vi "Arttu_v09_99.vi"() -> ()   [LabVIEW 2016]
uses:
  Desktop/Bertta-Bertta_deploy/Bertta-Bertta_deploy/BERTTA/x64/Debug/BERTTA.dll
panel:
  out "element":bool
  out "Started:":string
  in  "SHUTDOWN":bool
  in  "MASTER CONTROL":bool
  in  "Tab Control":T1(tab)
  out "Output File":path caption="selected path"
  in  "Browse folder":path=path "" caption="start path"
  in  "Read Seq":bool
  in  "Save Seq":bool
  in  "Configuration file":path=path "C:/Users/shresplab/Desktop/ArttuConfiguration.lvm" caption="Filename"
  in  "OK Button 2":bool
  out "Boolean":bool
  in  "User (initials)":string
  in  "Project name":string
  in  "Description":string
  out "PUMP1":bool
  out "Target amount":dbl
  out "Scale weight":dbl
  out "Amount now":dbl
  out "Flow rate":dbl
  out "Time to target":dbl format="%<%H:%M:%S>t"
  out "Current step":dbl
  out "Target":dbl
  out "Amount now":dbl
  out "Amount now":dbl
  out "Target":dbl
  out "Current step":dbl
  out "Time to target":dbl format="%<%H:%M:%S>t"
  out "Flow rate":dbl
  out "Amount now":dbl
  out "Scale weight":dbl
  out "Target amount":dbl
  out "PUMP2":bool
  out "Sensor OK 6":bool
  out "Sensor OK 5":bool
  out "Sensor OK 4":bool
  out "Sensor OK 3":bool
  in  "OK Button":bool
  in  "Add comment":string
  out "PUMP3":bool
  out "Target amount":dbl
  out "Scale weight":dbl
  out "Amount now":dbl
  out "Flow rate":dbl
  out "Time to target":dbl format="%<%H:%M:%S>t"
  out "Current step":dbl
  out "Target":dbl
  out "Amount now":dbl
  out "Tr":dbl
  out "Tj in":dbl
  out "Tj out":dbl
  out "T set":dbl
  out "Current step":i32
  out "RPM":dbl
  out "Torque 2":dbl
  out "Waveform Chart 5":dynamicdata(graph)
  out "Waveform Chart 6":dynamicdata(graph)
  out "Waveform Chart 7":dynamicdata(graph)
  in  "Tab Control 2":T2(tab)
  out "Waveform Chart 3":dynamicdata(graph)
  out "Waveform Chart 8":dynamicdata(graph)
  out "Waveform Chart 11":dynamicdata(graph)
  out "Waveform Chart 13":dynamicdata(graph)
  out "Waveform Chart 9":dynamicdata(graph)
  out "Table":string[][](table)=[["14.8.2017 18.06.59", "0,000000", "417,670000", "-0,150000", "1,000000", "22,220000", "23,366837", "23,574959", "23,985852", "23,690000", "240,000000", "4,000000", "0,000000", "397,000000", "-397,000000", "1,000000"], ["14.8.2017 18.07.06", "0,000000", "417,640000", "-0,120000", "1,000000", "22,220000", "23,763115", "23,906257", "23,985694", "23,680000", "240,000000", "4,000000", "0,000000", "397,000000", "-397,000000", "1,000000"], ["14.8.2017 18.07.13", "0,000000", "417,640000", "-0,120000", "1,000000", "22,220000", "23,965922", "24,013440", "23,984906", "23,670000", "240,000000", "4,100000", "3,000000", "397,000000", "-397,000000", "1,000000"], ["14.8.2017 18.07.21", "0,000000", "417,640000", "-0,120000", "1,000000", "22,220000", "23,943860", "23,900110", "23,987113", "23,670000", "240,000000", "4,000000", "0,000000", "397,000000", "-397,000000", "1,000000"], ["14.8.2017 18.07.28", "0,000000", "417,640000", "-0,120000", "1,000000", "22,220000", "23,736328", "23,600018", "23,989004", "23,660000", "240,000000", "4,000000", "0,000000", "397,000000", "-397,000000", "1,000000"], ["14.8.2017 18.07.36", "0,000000", "417,640000", "-0,120000", "1,000000", "22,220000", "23,480910", "23,324538", "23,991053", "23,660000", "240,000000", "4,000000", "0,000000", "397,000000", "-397,000000", "1,000000"], ["14.8.2017 18.07.43", "0,000000", "417,640000", "-0,120000", "2,000000", "22,220000", "23,195579", "23,008270", "23,999093", "23,650000", "240,000000", "4,000000", "0,000000", "397,000000", "-397,000000", "1,000000"], ["14.8.2017 18.07.51", "0,000000", "417,650000", "-417,650000", "1,000000", "22,220000", "22,862541", "22,649021", "24,003979", "23,650000", "240,000000", "4,000000", "0,000000", "397,000000", "-397,000000", "2,000000"], ["14.8.2017 18.07.58", "0,000000", "417,640000", "0,010000", "1,000000", "22,220000", "22,541353", "22,354878", "24,005398", "23,650000", "240,000000", "4,000000", "0,000000", "397,000000", "-397,000000", "1,000000"], ["14.8.2017 18.08.06", "0,000000", "417,640000", "0,010000", "1,000000", "22,220000", "22,347931", "22,253738", "24,007605", "23,640000", "240,000000", "4,100000", "0,000000", "397,000000", "-397,000000", "1,000000"], ["14.8.2017 18.08.13", "0,000000", "417,640000", "0,010000", "1,000000", "22,220000", "22,329030", "22,302102", "24,006028", "23,640000", "240,000000", "4,000000", "0,000000", "395,820000", "-395,820000", "1,000000"], ["14.8.2017 18.08.20", "0,000000", "417,640000", "0,010000", "1,000000", "22,220000", "22,466849", "22,511320", "24,002403", "23,630000", "240,000000", "4,000000", "0,000000", "395,830000", "-0,010000", "1,000000"], ["14.8.2017 18.08.28", "0,000000", "417,640000", "0,010000", "1,000000", "22,220000", "22,707062", "22,835101", "24,000984", "23,620000", "240,000000", "4,000000", "0,000000", "395,830000", "-0,010000", "1,000000"], ["14.8.2017 18.08.35", "0,000000", "417,640000", "0,010000", "1,000000", "22,220000", "23,054104", "23,232979", "24,001299", "23,600000", "240,000000", "4,000000", "0,000000", "395,830000", "-0,010000", "1,000000"], ["14.8.2017 18.08.43", "0,000000", "417,640000", "0,010000", "1,000000", "22,220000", "23,412371", "23,522793", "24,002560", "23,590000", "240,000000", "4,000000", "0,000000", "395,820000", "0,000000", "1,000000"], ["14.8.2017 18.08.51", "0,000000", "417,640000", "0,010000", "1,000000", "22,220000", "23,596247", "23,656125", "24,003821", "23,580000", "240,000000", "4,000000", "0,000000", "395,820000", "0,000000", "1,000000"]]
  in  "Manual/Ramp 3":bool=TRUE
  in  "Manual/Ramp 2":bool=TRUE
  out "Boolean 4":bool
  out "Boolean 3":bool
  out "Boolean 2":bool
  in  "Reset 6":bool
  in  "Manual/Ramp":bool=TRUE
  in  "Array":dbl[][](array[numeric])=[[20.0, 0.0], [20.0, 0.0], [20.0, 0.0]]
  in  "?":bool
  in  "Time":dbl format="Time to target (min):                %#_g"
  out "Current temp":dbl format="Current temperature (S1):   %#_6g"
  in  "OK Button 3":bool
  out "Sensor OK":bool
  in  "T fail":dbl=20.0 format="Failsafe temperature:              %#_g"
  in  "Setpoint":dbl=20.0 format="Temperature target:                %#_6g"
  out "Waveform Chart":dynamicdata(graph)
  out "T external 2":dbl format="Current temp (S2):    %#_g"
  in  "UPDATE TEMP":bool
  out "Led11 5":bool
  out "RPM":dbl format="%_4f"
  out "Led10 3":bool
  out "Led9 3":bool
  out "Led8 3":bool
  out "Led7 3":bool
  out "Led6 3":bool
  out "Led5 3":bool
  out "Led4 3":bool
  out "Led3 3":bool
  out "Led2 3":bool
  out "Led1 3":bool
  in  "PumpSeq 4":dbl[][](array[numeric])=[[0.0, 0.0, 0.0, 0.0, 0.0, 0.0, 0.0, 0.0, 0.0, 0.0], [0.0, 0.0, 0.0, 0.0, 0.0, 0.0, 0.0, 0.0, 0.0, 0.0], [0.0, 0.0, 0.0, 0.0, 0.0, 0.0, 0.0, 0.0, 0.0, 0.0], [0.0, 0.0, 0.0, 0.0, 0.0, 0.0, 0.0, 0.0, 0.0, 0.0], [0.0, 0.0, 0.0, 0.0, 0.0, 0.0, 0.0, 0.0, 0.0, 0.0], [0.0, 0.0, 0.0, 0.0, 0.0, 0.0, 0.0, 0.0, 0.0, 0.0], [0.0, 0.0, 0.0, 0.0, 0.0, 0.0, 0.0, 0.0, 0.0, 0.0], [0.0, 0.0, 0.0, 0.0, 0.0, 0.0, 0.0, 0.0, 0.0, 0.0], [0.0, 0.0, 0.0, 0.0, 0.0, 0.0, 0.0, 0.0, 0.0, 0.0], [0.0, 0.0, 0.0, 0.0, 0.0, 0.0, 0.0, 0.0, 0.0, 0.0]]
  in  "?":bool
  out "Flow rate (g/min)":dbl
  out "Scale reading":dbl
  out "Step amount now":dbl
  in  "Grams / min":dbl
  out "Waveform Chart 14":dynamicdata(graph)
  in  "?":bool
  out "Total amount now":dbl
  out "Led11 4":bool
  in  "Reset 5":bool
  out "Elapsed / step":i32
  out "Time to target":dbl format="%<%H:%M:%S>t"
  in  "OK Button 4":bool
  out "Led11":bool
  out "RPM":dbl format="%_4f"
  out "Led10":bool
  out "Led9":bool
  out "Led8":bool
  out "Led7":bool
  out "Led6":bool
  out "Led5":bool
  out "Led4":bool
  out "Led3":bool
  out "Led2":bool
  out "Led1":bool
  in  "PumpSeq 2":dbl[][](array[numeric])=[[0.0, 0.0, 0.0, 0.0, 0.0, 0.0, 0.0, 0.0, 0.0, 0.0], [0.0, 0.0, 0.0, 0.0, 0.0, 0.0, 0.0, 0.0, 0.0, 0.0], [0.0, 0.0, 0.0, 0.0, 0.0, 0.0, 0.0, 0.0, 0.0, 0.0], [0.0, 0.0, 0.0, 0.0, 0.0, 0.0, 0.0, 0.0, 0.0, 0.0], [0.0, 0.0, 0.0, 0.0, 0.0, 0.0, 0.0, 0.0, 0.0, 0.0], [0.0, 0.0, 0.0, 0.0, 0.0, 0.0, 0.0, 0.0, 0.0, 0.0], [0.0, 0.0, 0.0, 0.0, 0.0, 0.0, 0.0, 0.0, 0.0, 0.0], [0.0, 0.0, 0.0, 0.0, 0.0, 0.0, 0.0, 0.0, 0.0, 0.0], [0.0, 0.0, 0.0, 0.0, 0.0, 0.0, 0.0, 0.0, 0.0, 0.0], [0.0, 0.0, 0.0, 0.0, 0.0, 0.0, 0.0, 0.0, 0.0, 0.0]]
  in  "?":bool
  out "Flow rate (g/min)":dbl
  out "Scale reading":dbl
  out "Step amount now":dbl
  in  "Grams / min":dbl
  out "Waveform Chart 10":dynamicdata(graph)
  in  "?":bool
  out "Total amount now":dbl
  out "Led11":bool
  in  "Reset 3":bool
  out "Elapsed / step":i32
  out "Time to target":dbl format="%<%H:%M:%S>t"
  in  "OK Button 5":bool
  out "Led11 3":bool
  out "RPM":dbl format="%_4f"
  out "Led10 2":bool
  out "Led9 2":bool
  out "Led8 2":bool
  out "Led7 2":bool
  out "Led6 2":bool
  out "Led5 2":bool
  out "Led4 2":bool
  out "Led3 2":bool
  out "Led2 2":bool
  out "Led1 2":bool
  in  "PumpSeq 3":dbl[][](array[numeric])=[[0.0, 0.0, 0.0, 0.0, 0.0, 0.0, 0.0, 0.0, 0.0, 0.0], [0.0, 0.0, 0.0, 0.0, 0.0, 0.0, 0.0, 0.0, 0.0, 0.0], [0.0, 0.0, 0.0, 0.0, 0.0, 0.0, 0.0, 0.0, 0.0, 0.0], [0.0, 0.0, 0.0, 0.0, 0.0, 0.0, 0.0, 0.0, 0.0, 0.0], [0.0, 0.0, 0.0, 0.0, 0.0, 0.0, 0.0, 0.0, 0.0, 0.0], [0.0, 0.0, 0.0, 0.0, 0.0, 0.0, 0.0, 0.0, 0.0, 0.0], [0.0, 0.0, 0.0, 0.0, 0.0, 0.0, 0.0, 0.0, 0.0, 0.0], [0.0, 0.0, 0.0, 0.0, 0.0, 0.0, 0.0, 0.0, 0.0, 0.0], [0.0, 0.0, 0.0, 0.0, 0.0, 0.0, 0.0, 0.0, 0.0, 0.0], [0.0, 0.0, 0.0, 0.0, 0.0, 0.0, 0.0, 0.0, 0.0, 0.0]]
  in  "?":bool
  out "Flow rate (g/min)":dbl
  out "Scale reading":dbl
  out "Step amount now":dbl
  in  "Grams / min":dbl
  out "Waveform Chart 12":dynamicdata(graph)
  in  "?":bool
  out "Total amount now":dbl
  out "Led11 2":bool
  in  "Reset 4":bool
  out "Elapsed / step":i32
  out "Time to target":dbl format="%<%H:%M:%S>t"
  in  "OK Button 6":bool
  in  "?":bool
  in  "Scale port":dbl=3.0
  out "Waveform Chart 15":dynamicdata(graph)
  in  "?":bool
  in  "OK Button 8":bool
  in  "Remote / Manual":bool
  in  "Set RPM":i32
  out "RPM":dbl
  out "Torque":dbl
  out "Waveform Chart 4":dynamicdata(graph)
  in  "OK Button 7":bool
  out "PortDev out":dbl[](array[numeric])
  in  "Save PortDev":bool
  out "PortDev in":dbl[](array[numeric])
  in  "dev1":i32=1
  in  "dev2":i32=2
  in  "dev3":i32=3
  in  "dev4":i32=4
  in  "dev5":i32=5
  in  "dev6":i32=5
  in  "dev8":i32
  in  "port1":i32=7
  in  "port2":i32=7
  in  "port3":i32=2
  in  "port4":i32=2
  in  "port5":i32=5
  in  "port6":i32=4
  in  "port7":i32=3
  in  "port8":i32
  in  "dev7":i32=5
  in  "Treshold (T/C)":dbl=0.5
  out "DAQ 9217 (PT100)":errorcluster
  out "Config File":dbl[][](array[numeric])
  in  "Temp Control":tag="cDAQ9188XT-1C3BEFEMod1"
  in  "PAM Control":tag="cDAQ9188XT-1C3BEFEMod7"
  # "Temperature sensor:"
  # "Manual control:"
  # "PUMP & SCALE 1"
  # "STEP"
  # "TOTAL"
  # "PUMP & SCALE 2"
  # "STEP"
  # "TOTAL"
  # "PUMP & SCALE 3"
  # "STEP"
  # "TOTAL"
  # "Temperature control parameter"
  # "Secondary temperature sensor"
  # "Temp target"
  # "Time target"
  # "Grams    /   min"
  # "End of sequence"
  # "Manual control"
  # "Grams    /   min"
  # "End of sequence"
  # "Manual control"
  # "Grams    /   min"
  # "End of sequence"
  # "Manual control"
  # "PAM control"
  # "dev1 and dev2 always to port1 and 2\nport1 = port2 = Lauda\n\ndev3 and dev4 always to port3 and port4\nport3 = port4 = Heidolph"
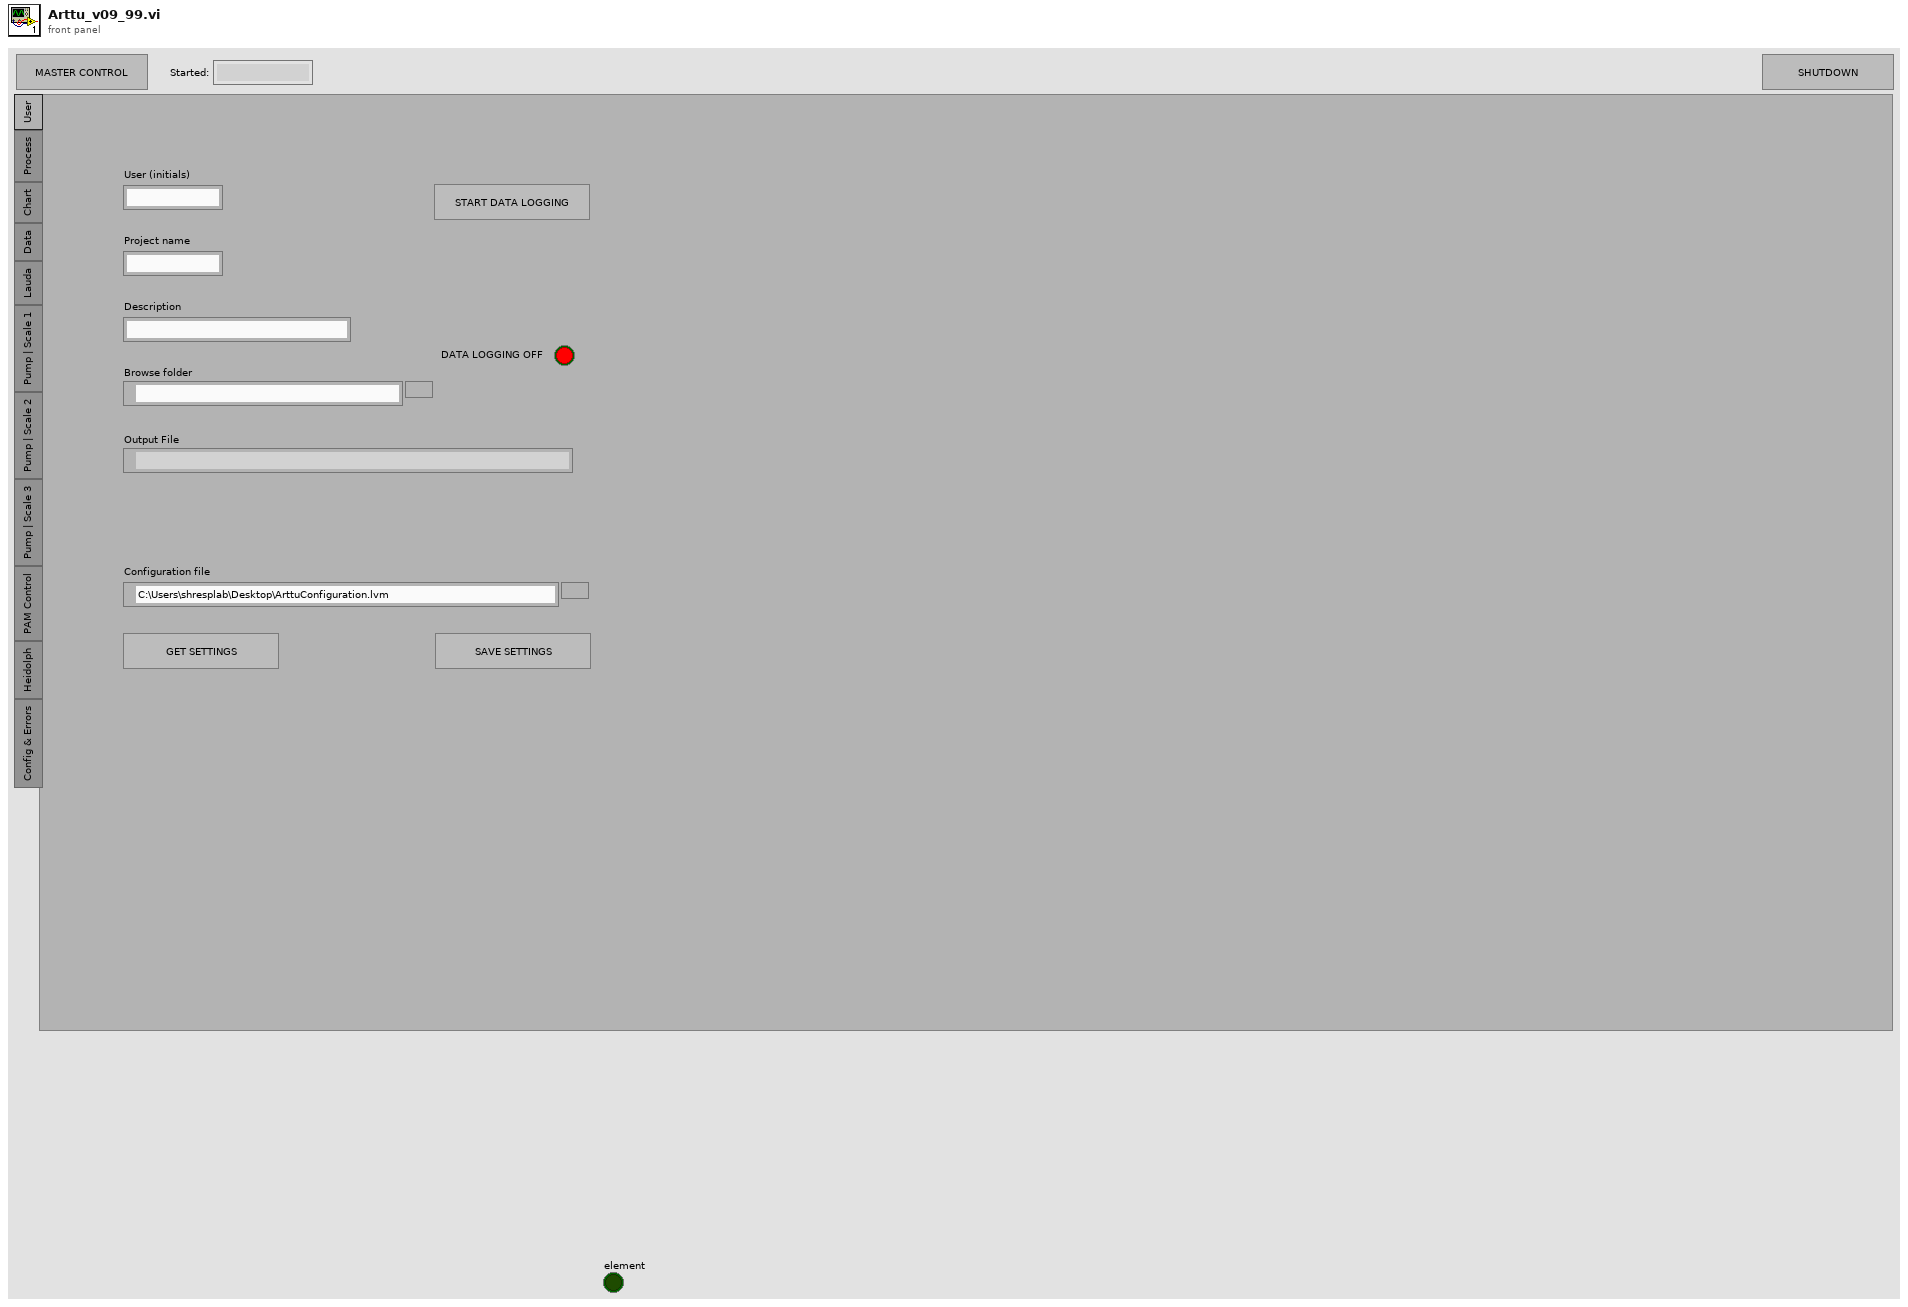
[diagram p1: front panel]
types:
  T1 = enum32{"User", "Process", "Chart", "Data", "Lauda", "Pump | Scale 1", "Pump | Scale 2", "Pump | Scale 3", "PAM Control", "Heidolph", "Config & Errors"}
  T2 = enum32{"Temperatures", "Scale / Pump 1", "Scale / Pump 2", "Scale / Pump 3", "RPM / torque"}
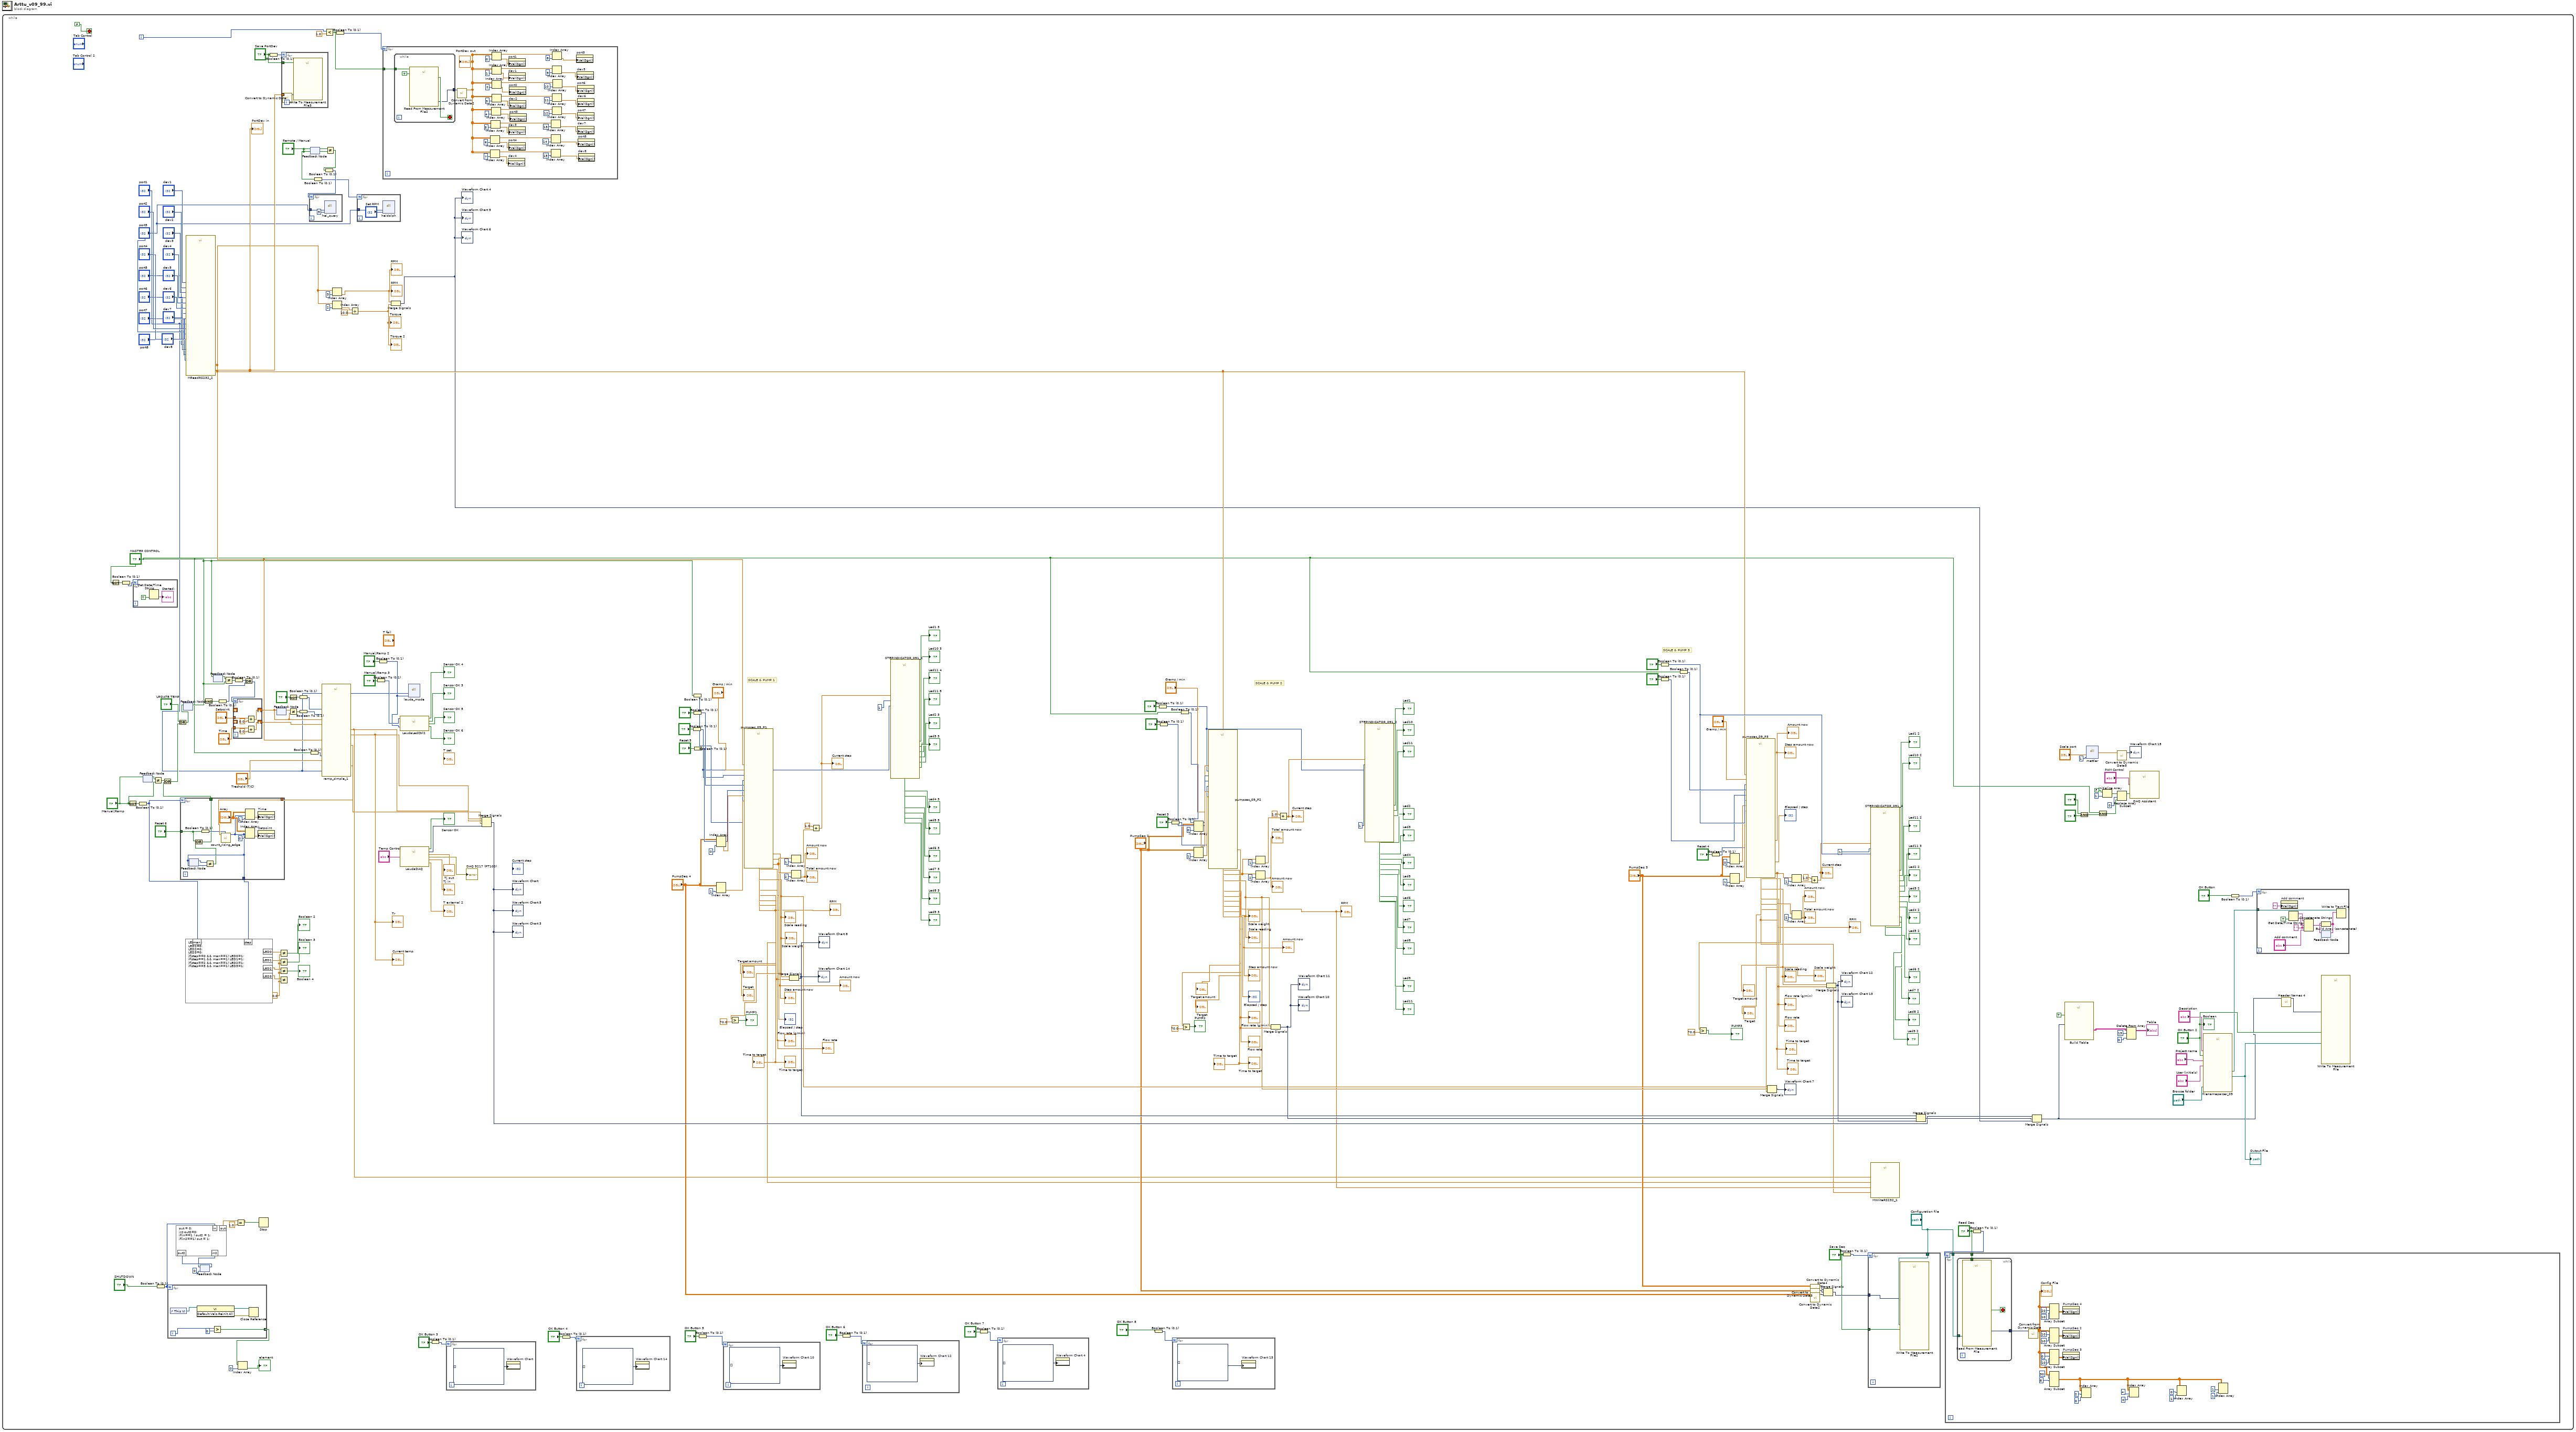
[diagram p0: block diagram]
diagram:
  n1 = while {
    i -> [w65]
    stop <- FALSE stop-if-true
    w51 = 0.0 ("y")
    # "SCALE & PUMP 1"
    # "SCALE & PUMP 3"
    # "SCALE & PUMP 2"
    n2 = Not(x="MASTER CONTROL") -> (.not. x?=w292:bool)
    n3 = Boolean To (0,1)(Boolean=w292) -> (0, 1=w293:i16)
    n4 = Not(x="Manual/Ramp") -> (.not. x?=w58:bool)
    n5 = for {
      N: w293 -> [_]
      n6 = Get Date/Time String(want seconds? (F)=TRUE) -> (time string=→"Started:":string)  [unwired: 2 in, 1 out]
    }
    n7 = Boolean To (0,1)(Boolean=w58) -> (0, 1=w40:i16)
    n8 = feedback #1() -> (w46:bool)  [unwired: 1 in]
    n9 = feedback-in #1("Manual/Ramp") -> ()
    n10 = Not Equal?(x=w46, y="Manual/Ramp") -> (x != y?=w43:bool)
    n11 = Boolean To (0,1)(Boolean="SHUTDOWN") -> (0, 1=w277:i16)
    n12 = for {
      N: w277 -> [_]
      tunnel: [w409] -> w291 mode=indexing
      i -> [w411]
      n13 = control-ref of="This VI"() -> (w414:refnum<vi>)
      n14 = invoke class="VI" method="Default Vals.Reinit All"(reference=w414) -> (reference out=w412:refnum<vi>, error out=w413:errorcluster)  [unwired: 2 in, 1 out]
      n15 = Greater?(x=w411, y=0) -> (0:w409:bool)
      n16 = Close Reference(reference=w412, error in (no error)=w413) -> ()  [unwired: 1 out]
    }
    n17 = feedback #2() -> (w38:bool)  [unwired: 1 in]
    n18 = call "MReadRS232_2.vi"("port1"="port1", "dev1"="dev1", "port2"="port2", "dev2"="dev2", "port3"="port3", "dev7"="dev7", "dev8"="dev8", "port7"="port7", "port8"="port8", "dev5"="dev5", "port5"="port5", "dev4"="dev4", "dev6"="dev6", "port6"="port6", "port4"="port4", "dev3"="dev3") -> ("output array"=w69:dbl[], "params"=w30:dbl[])  [unwired: 2 in]
    "PortDev in" <- w69
    n19 = feedback #3(0) -> (w275:i32)
    n20 = formula code="out = 0;\nint out2=0;\nif(in==1 ) out2 = 1;\nif(in2==1) out = 1;"("in"=w277, "in2"=w275) -> ("out"=w279:dbl, "out2"=w276:i32)
    n21 = feedback-in #3(w276) -> ()
    n22 = And(x="MASTER CONTROL", y=w38) -> (x .and. y?=w96:bool)
    n23 = feedback #4() -> (w87:bool)  [unwired: 1 in]
    n24 = feedback-in #4("MASTER CONTROL") -> ()
    n25 = Boolean To (0,1)(Boolean=w96) -> (0, 1=w85:i16)
    n26 = Not Equal?(x=w87, y="MASTER CONTROL") -> (x != y?=w86:bool)
    n27 = Boolean To (0,1)(Boolean=w86) -> (0, 1=w84:i16)
    n28 = Equal?(x=w279, y=1.0) -> (x = y?=w278:bool)
    n29 = Index Array(array=w291, index=0) -> (element=→"element":bool)
    n30 = Or(x=w84, y=w85) -> (x .or. y?=w83:i16)
    n31 = for {
      N: w83 -> [_]
      tunnel: "Time" -> [w361]
      shift-right: [w360] -> w97
      shift-left: _ -> [_]
      tunnel: "Setpoint" -> [w358]
      shift-right: [w357] -> w94
      shift-left: _ -> [_]
      n32 = Add(x=w358, y=0.0) -> (x+y=w357:dbl)
      n33 = Add(x=w361, y=0.0) -> (x+y=w360:dbl)
    }
    n34 = Stop(stop? (T)=w278) -> ()
    n35 = Boolean To (0,1)(Boolean="Save PortDev") -> (0, 1=w68:i16)
    n36 = feedback-in #5(w94) -> ()
    n37 = feedback #5() -> (w95:dbl)  [unwired: 1 in]
    n38 = for {
      N: w68 -> [_]
      tunnel: w69 -> [w356]
      tunnel: "Save PortDev" -> [w354]
      n39 = call "Convert to Dynamic Data"("Array"=w356) -> ("Dynamic Data Type"=w355:dynamicdata)  [unwired: 3 in]
      n40 = call "Write To Measurement File3"("Signals"=w355, "Reset"=w354) -> ()  [unwired: 15 in, 3 out]
    }
    n41 = Not(x="?") -> (.not. x?=w90:bool)
    n42 = Not Equal?(x=w95, y=w94) -> (x != y?=w93:bool)
    n43 = Boolean To (0,1)(Boolean=w90) -> (0, 1=w92:i16)
    n44 = Boolean To (0,1)(Boolean=w93) -> (0, 1=w88:i16)
    n45 = Boolean To (0,1)(Boolean="MASTER CONTROL") -> (0, 1=w89:i16)
    n46 = feedback-in #6("Remote / Manual") -> ()
    n47 = feedback #6() -> (w35:bool)  [unwired: 1 in]
    n48 = Boolean To (0,1)(Boolean="Remote / Manual") -> (0, 1=w33:i16)
    n49 = call "ramp_simple_1.vi"("pause"=w92, "time_set"=w97, "array"=w30, "reset"=w88, "master"=w89, "T_sp"=w94, "treshold"="Treshold (T/C)", "port"="port1") -> ("Tin"=w100:dbl, "Tr"=w101:dbl, "target_reached"=w56:dbl, "T control"=w102:dbl)  [unwired: 3 in, 1 out]
    "Tr" <- w101
    "Current temp" <- w101
    n50 = for {
      N: w40 -> [_]
      tunnel: w56 -> [w313]
      tunnel: [w303] -> w44
      tunnel: "Reset 6" -> [w305]
      tunnel: [w306] -> w47
      n51 = feedback #7() -> (w307:i32)  [unwired: 1 in]
      n52 = Boolean To (0,1)(Boolean=w305) -> (0, 1=w308:i16)
      n53 = call "count_rising_edge.vi"("reset"=w308, "target_reached"=w313) -> ("element 2"=w306:i32)  [unwired: 9 in]
      n54 = feedback-in #7(w306) -> ()
      n55 = Not Equal?(x=w307, y=w306) -> (x != y?=w304:bool)
      n56 = Or(x=w305, y=w304) -> (x .or. y?=w303:bool)
      n57 = Index Array(array="Array", index (row)=w306, index (col)=1 ("disabled index (col)")) -> (element=w309:dbl)
      n58 = Index Array(array="Array", index (row)=w306, index (col)=0 ("disabled index (col)")) -> (element=w310:dbl)
      n59 = property on="Time" class="DigNum (strict)"("Val(Sgnl)"=w309) -> ()  [unwired: 2 in, 2 out]
      n60 = property on="Setpoint" class="DigNum (strict)"("Val(Sgnl)"=w310) -> ()  [unwired: 2 in, 2 out]
    }
    n61 = Or(x=w43, y=w44) -> (x .or. y?=w42:bool)
    n62 = Or(x="UPDATE TEMP", y=w42) -> (x .or. y?=w39:bool)
    n63 = feedback-in #2(w39) -> ()
    n64 = formula code="LED0=0;\nLED1=0;\nLED2=0;\nLED3=0;\nif(step==0 && man==1) LED0=1;\nif(step==1 && man==1) LED1=1;\nif(step==2 && man==1) LED2=1;\nif(step==3 && man==1) LED3=1;"("step"=w47, "man"=w40) -> ("LED0"=w55:dbl, "LED1"=w54:dbl, "LED2"=w53:dbl, "LED3"=w52:dbl)
    n65 = Not Equal?(x=w55, y=w51) -> (x != y?=→"Boolean 2":bool)
    n66 = Not Equal?(x=w54, y=w51) -> (x != y?=→"Boolean 3":bool)
    n67 = Not Equal?(x=w53, y=w51) -> (x != y?=→"Boolean 4":bool)
    n68 = Not Equal?(x=w52, y=w51) -> ()  [unwired: 1 out]
    n69 = Less?(x=w65, y=1.0) -> (x < y?=w63:bool)
    n70 = Not Equal?(x=w35, y="Remote / Manual") -> (x != y?=w34:bool)
    n71 = Boolean To (0,1)(Boolean=w34) -> (0, 1=w36:i16)
    n72 = for {
      N: w36 -> [_]
      tunnel: "port3" -> [w301]
      n73 = dll-call lib="C:/Users/shresplab/Desktop/Bertta-Bertta_deploy/Bertta-Bertta_deploy/BERTTA/x64/Debug/BERTTA.dll" fn="hei_query"("port"=w301, "q"=5) -> ()  [unwired: 6 in, 2 out]
    }
    n74 = Index Array(array=w30, index=3) -> (element=w27:dbl)
    "RPM" <- w27
    "RPM" <- w27
    n75 = Index Array(array=w30, index=2) -> (element=w29:dbl)
    n76 = Boolean To (0,1)(Boolean=w63) -> (0, 1=w64:i16)
    n77 = Divide(x=w29, y=10.0) -> (x/y=w26:dbl)
    "Torque" <- w26
    "Torque 2" <- w26
    n78 = for {
      N: w33 -> [_]
      tunnel: "port3" -> [w299]
      n79 = dll-call lib="C:/Users/shresplab/Desktop/Bertta-Bertta_deploy/Bertta-Bertta_deploy/BERTTA/x64/Debug/BERTTA.dll" fn="heidolph"("port"=w299, "speed"="Set RPM") -> ()  [unwired: 6 in, 2 out]
    }
    n80 = Boolean To (0,1)(Boolean="Manual/Ramp 3") -> (0, 1=w3:i16)
    n81 = Boolean To (0,1)(Boolean="Manual/Ramp 2") -> (0, 1=w1:i16)
    n82 = for {
      N: w64 -> [_]
      tunnel: w63 -> [w349]
      n83 = while {
        tunnel: [w352] -> w348
        tunnel: w349 -> [w350]
        stop <- w353 stop-if-true
        n84 = call "Read From Measurement File2"("Enable"=TRUE, "Reset"=w350) -> ("Signals"=w352:dynamicdata, "EOF?"=w353:bool)  [unwired: 4 in, 4 out]
      }
      n85 = call "Convert from Dynamic Data2"("Dynamic Data Type"=w348) -> ("Array"=w331:dbl[])  [unwired: 3 in]
      "PortDev out" <- w331
      n86 = Index Array(array=w331, index=6) -> (element=w324:dbl)
      n87 = Index Array(array=w331, index=7) -> (element=w323:dbl)
      n88 = Index Array(array=w331, index=5) -> (element=w325:dbl)
      n89 = Index Array(array=w331, index=4) -> (element=w326:dbl)
      n90 = Index Array(array=w331, index=0) -> (element=w330:dbl)
      n91 = Index Array(array=w331, index=1) -> (element=w329:dbl)
      n92 = Index Array(array=w331, index=3) -> (element=w327:dbl)
      n93 = Index Array(array=w331, index=2) -> (element=w328:dbl)
      n94 = property on="dev4" class="DigNum (strict)"("Val(Sgnl)"=w323) -> ()  [unwired: 2 in, 2 out]
      n95 = property on="dev3" class="DigNum (strict)"("Val(Sgnl)"=w325) -> ()  [unwired: 2 in, 2 out]
      n96 = property on="port4" class="DigNum (strict)"("Val(Sgnl)"=w324) -> ()  [unwired: 2 in, 2 out]
      n97 = property on="port1" class="DigNum (strict)"("Val(Sgnl)"=w330) -> ()  [unwired: 2 in, 2 out]
      n98 = property on="dev1" class="DigNum (strict)"("Val(Sgnl)"=w329) -> ()  [unwired: 2 in, 2 out]
      n99 = property on="port2" class="DigNum (strict)"("Val(Sgnl)"=w328) -> ()  [unwired: 2 in, 2 out]
      n100 = property on="dev2" class="DigNum (strict)"("Val(Sgnl)"=w327) -> ()  [unwired: 2 in, 2 out]
      n101 = property on="port3" class="DigNum (strict)"("Val(Sgnl)"=w326) -> ()  [unwired: 2 in, 2 out]
      n102 = Index Array(array=w331, index=14) -> (element=w316:dbl)
      n103 = Index Array(array=w331, index=15) -> (element=w315:dbl)
      n104 = Index Array(array=w331, index=13) -> (element=w317:dbl)
      n105 = Index Array(array=w331, index=12) -> (element=w318:dbl)
      n106 = Index Array(array=w331, index=8) -> (element=w322:dbl)
      n107 = Index Array(array=w331, index=9) -> (element=w321:dbl)
      n108 = Index Array(array=w331, index=11) -> (element=w319:dbl)
      n109 = Index Array(array=w331, index=10) -> (element=w320:dbl)
      n110 = property on="port5" class="DigNum (strict)"("Val(Sgnl)"=w322) -> ()  [unwired: 2 in, 2 out]
      n111 = property on="dev5" class="DigNum (strict)"("Val(Sgnl)"=w321) -> ()  [unwired: 2 in, 2 out]
      n112 = property on="port6" class="DigNum (strict)"("Val(Sgnl)"=w320) -> ()  [unwired: 2 in, 2 out]
      n113 = property on="dev6" class="DigNum (strict)"("Val(Sgnl)"=w319) -> ()  [unwired: 2 in, 2 out]
      n114 = property on="port7" class="DigNum (strict)"("Val(Sgnl)"=w318) -> ()  [unwired: 2 in, 2 out]
      n115 = property on="dev7" class="DigNum (strict)"("Val(Sgnl)"=w317) -> ()  [unwired: 2 in, 2 out]
      n116 = property on="port8" class="DigNum (strict)"("Val(Sgnl)"=w316) -> ()  [unwired: 2 in, 2 out]
      n117 = property on="dev8" class="DigNum (strict)"("Val(Sgnl)"=w315) -> ()  [unwired: 2 in, 2 out]
    }
    n118 = Merge Signals(w27, w26) -> (w25:dynamicdata)
    "Waveform Chart 4" <- w25
    "Waveform Chart 6" <- w25
    "Waveform Chart 9" <- w25
    n119 = call "LaudaLedCtrl2.vi"("ctrl_mode"=w1, "T ext / T ext in"=w3) -> ("Sensor OK 5"=→"Sensor OK 5":bool, "Sensor OK 3"=→"Sensor OK 3":bool, "Sensor OK 4"=→"Sensor OK 4":bool, "Sensor OK 6"=→"Sensor OK 6":bool)  [unwired: 6 in]
    n120 = call "LaudaDAQ.vi"("device name"="Temp Control") -> ("error out"=→"DAQ 9217 (PT100)":errorcluster, 1:"Tj out"=→"Tj out":dbl, "data"=w169:dynamicdata, "Sensor OK"=→"Sensor OK":bool, 4:"Tj out"=→"Tj in":dbl, "T external 2"=→"T external 2":dbl)  [unwired: 5 in]
    n121 = dll-call lib="C:/Users/shresplab/Desktop/Bertta-Bertta_deploy/Bertta-Bertta_deploy/BERTTA/x64/Debug/BERTTA.dll" fn="lauda_mode"("port"="port1", "mode"=w1) -> ()  [unwired: 6 in, 2 out]
    n122 = Boolean To (0,1)(Boolean="OK Button 3") -> (0, 1=w113:i16)
    n123 = for {
      N: w113 -> [_]
      n124 = property on="Waveform Chart" class="WFChart (strict)"("History Data"=dynamicdata[] []) -> ()  [unwired: 2 in, 2 out]
    }
    n125 = Merge Signals(w102, w101, w100, w169) -> (w170:dynamicdata)
    "Waveform Chart 3" <- w170
    "Waveform Chart" <- w170
    "Waveform Chart 5" <- w170
    n126 = Boolean To (0,1)(Boolean="OK Button 4") -> (0, 1=w111:i16)
    n127 = for {
      N: w111 -> [_]
      n128 = property on="Waveform Chart 14" class="WFChart (strict)"("History Data"=dynamicdata[] []) -> ()  [unwired: 2 in, 2 out]
    }
    n129 = Boolean To (0,1)(Boolean="?") -> (0, 1=w178:i16)
    n130 = Boolean To (0,1)(Boolean="?") -> (0, 1=w182:i16)
    n131 = Boolean To (0,1)(Boolean="MASTER CONTROL") -> (0, 1=w174:i16)
    n132 = Boolean To (0,1)(Boolean="Reset 5") -> (0, 1=w181:i16)
    n133 = Boolean To (0,1)(Boolean="OK Button 5") -> (0, 1=w109:i16)
    n134 = Index Array(array="PumpSeq 4", index (col)=0) -> (element=w186:dbl[])  [unwired: 1 in]
    n135 = Index Array(array="PumpSeq 4", index (col)=1) -> (element=w207:dbl[])  [unwired: 1 in]
    n136 = for {
      N: w109 -> [_]
      n137 = property on="Waveform Chart 10" class="WFChart (strict)"("History Data"=dynamicdata[] []) -> ()  [unwired: 2 in, 2 out]
    }
    n138 = call "pumpsec_09_P1.vi"("reset"=w181, "master"=w174, "manual"=w178, "pause"=w182, "Array"=w30, "Target"=w186, "fr_manual"="Grams / min", "Time"=w207) -> ("pumpCtrl"=w153:dbl, "totaltarget"=→"Target":dbl, "target_step"=→"Target amount":dbl, "REGLO D"=w119:dbl, "time_to_target"=→"Time to target" →"Time to target":dbl, "step_fr"=w130:dbl, "amount_step"=→"Amount now" →"Step amount now":dbl, "Scale"=w165:dbl, "elapsed_step"=→"Elapsed / step":dbl, "params"=w204:dbl[])  [unwired: 8 in, 2 out]
    "Flow rate" <- w130
    "Scale weight" <- w165
    "Scale reading" <- w165
    "Flow rate (g/min)" <- w130
    "RPM" <- w119
    n139 = Greater?(x=w153, y=70.0) -> (0:→"PUMP1":bool)
    n140 = Merge Signals(w165, w130) -> (w173:dynamicdata)
    "Waveform Chart 8" <- w173
    "Waveform Chart 14" <- w173
    n141 = Index Array(array=w204, index=1) -> (element=w201:dbl)
    n142 = Index Array(array=w204, index=2) -> (element=→"Amount now" →"Total amount now":dbl)
    n143 = Add(x=1.0, y=w201) -> (x+y=w131:dbl)
    "Current step" <- w131
    n144 = Boolean To (0,1)(Boolean="OK Button 6") -> (0, 1=w107:i16)
    n145 = for {
      N: w107 -> [_]
      n146 = property on="Waveform Chart 12" class="WFChart (strict)"("History Data"=dynamicdata[] []) -> ()  [unwired: 2 in, 2 out]
    }
    n147 = call "STEPINDICATOR_091_2.vi"("current step"=w131, "enable"=i16 1, "manual"=w178) -> ("Led 8"=→"Led8 3":bool, "Led 10"=→"Led10 3":bool, "Led 11"=→"Led11 4":bool, "Led 7"=→"Led7 3":bool, "Led 1"=→"Led1 3":bool, "Led 6"=→"Led6 3":bool, "Led 2"=→"Led2 3":bool, "Led 12"=→"Led11 5":bool, "Led 5"=→"Led5 3":bool, "Led 4"=→"Led4 3":bool, "Led 3"=→"Led3 3":bool, "Led 9"=→"Led9 3":bool)  [unwired: 1 in]
    n148 = Boolean To (0,1)(Boolean="OK Button 7") -> (0, 1=w105:i16)
    n149 = for {
      N: w105 -> [_]
      n150 = property on="Waveform Chart 4" class="WFChart (strict)"("History Data"=dynamicdata[] []) -> ()  [unwired: 2 in, 2 out]
    }
    n151 = Boolean To (0,1)(Boolean="OK Button 8") -> (0, 1=w22:i16)
    n152 = Boolean To (0,1)(Boolean="?") -> (0, 1=w241:i16)
    n153 = Boolean To (0,1)(Boolean="?") -> (0, 1=w267:i16)
    n154 = Boolean To (0,1)(Boolean="Reset 3") -> (0, 1=w265:i16)
    n155 = for {
      N: w22 -> [_]
      n156 = property on="Waveform Chart 15" class="WFChart (strict)"("History Data"=dynamicdata[] []) -> ()  [unwired: 2 in, 2 out]
    }
    n157 = Boolean To (0,1)(Boolean="MASTER CONTROL") -> (0, 1=w259:i16)
    n158 = Index Array(array="PumpSeq 2", index (col)=0 ("disabled index (col)")) -> (element=w270:dbl[])  [unwired: 1 in]
    n159 = Index Array(array="PumpSeq 2", index (col)=1 ("disabled index (col)")) -> (element=w269:dbl[])  [unwired: 1 in]
    n160 = call "pumpsec_09_P2.vi"("reset"=w265, "master"=w259, "manual"=w241, "pause"=w267, "Array"=w30, "Target"=w270, "fr_manual"="Grams / min", "Time"=w269) -> ("pumpCtrl"=w149:dbl, "totaltarget"=→"Target":dbl, "target_step"=→"Target amount":dbl, "REGLO D"=w118:dbl, "time_to_target"=→"Time to target" →"Time to target":dbl, "step_fr"=w168:dbl, "amount_step"=→"Amount now" →"Step amount now":dbl, "Scale"=w164:dbl, "elapsed_step"=→"Elapsed / step":dbl, "params"=w260:dbl[])  [unwired: 8 in, 2 out]
    "Scale weight" <- w164
    "Flow rate" <- w168
    "Scale reading" <- w164
    "Flow rate (g/min)" <- w168
    "RPM" <- w118
    n161 = Greater?(x=w149, y=70.0) -> (0:→"PUMP2":bool)
    n162 = Index Array(array=w260, index=1) -> (element=w263:dbl)
    n163 = Index Array(array=w260, index=2) -> (element=→"Amount now" →"Total amount now":dbl)
    n164 = Merge Signals(w164, w168) -> (w175:dynamicdata)
    "Waveform Chart 11" <- w175
    "Waveform Chart 10" <- w175
    n165 = Add(x=1.0, y=w263) -> (x+y=w257:dbl)
    "Current step" <- w257
    n166 = call "STEPINDICATOR_091_2.vi"("current step"=w257, "enable"=i16 1, "manual"=w241) -> ("Led 8"=→"Led8":bool, "Led 10"=→"Led10":bool, "Led 11"=→"Led11":bool, "Led 7"=→"Led7":bool, "Led 1"=→"Led1":bool, "Led 6"=→"Led6":bool, "Led 2"=→"Led2":bool, "Led 12"=→"Led11":bool, "Led 5"=→"Led5":bool, "Led 4"=→"Led4":bool, "Led 3"=→"Led3":bool, "Led 9"=→"Led9":bool)  [unwired: 1 in]
    n167 = Boolean To (0,1)(Boolean="?") -> (0, 1=w235:i16)
    n168 = Boolean To (0,1)(Boolean="?") -> (0, 1=w234:i16)
    n169 = Boolean To (0,1)(Boolean="MASTER CONTROL") -> (0, 1=w236:i16)
    n170 = Boolean To (0,1)(Boolean="Reset 4") -> (0, 1=w216:i16)
    n171 = Index Array(array="PumpSeq 3", index (col)=0 ("disabled index (col)")) -> (element=w219:dbl[])  [unwired: 1 in]
    n172 = Index Array(array="PumpSeq 3", index (col)=1 ("disabled index (col)")) -> (element=w218:dbl[])  [unwired: 1 in]
    n173 = call "pumpsec_09_P3.vi"("reset"=w216, "master"=w236, "manual"=w235, "pause"=w234, "Array"=w30, "Target"=w219, "fr_manual"="Grams / min", "Time"=w218) -> ("pumpCtrl"=w146:dbl, "totaltarget"=→"Target":dbl, "target_step"=→"Target amount":dbl, "REGLO D"=w117:dbl, "time_to_target"=→"Time to target" →"Time to target":dbl, "step_fr"=w167:dbl, "amount_step"=→"Amount now" →"Step amount now":dbl, "Scale"=w163:dbl, "elapsed_step"=→"Elapsed / step":dbl, "params"=w209:dbl[])  [unwired: 8 in, 2 out]
    "Scale weight" <- w163
    "Flow rate" <- w167
    "Scale reading" <- w163
    "Flow rate (g/min)" <- w167
    "RPM" <- w117
    n174 = Greater?(x=w146, y=70.0) -> (0:→"PUMP3":bool)
    n175 = Merge Signals(w165, w164, w163) -> (→"Waveform Chart 7":dynamicdata)
    n176 = Index Array(array=w209, index=1) -> (element=w210:dbl)
    n177 = Index Array(array=w209, index=2) -> (element=→"Amount now" →"Total amount now":dbl)
    n178 = Add(x=1.0, y=w210) -> (x+y=w208:dbl)
    "Current step" <- w208
    n179 = call "Convert to Dynamic Data4"("2D Array"="PumpSeq 3") -> ("Dynamic Data Type"=w122:dynamicdata)  [unwired: 3 in]
    n180 = call "Convert to Dynamic Data3"("2D Array"="PumpSeq 2") -> ("Dynamic Data Type"=w124:dynamicdata)  [unwired: 3 in]
    n181 = call "Convert to Dynamic Data2"("2D Array"="PumpSeq 4") -> ("Dynamic Data Type"=w127:dynamicdata)  [unwired: 3 in]
    n182 = Merge Signals(w122, w124, w127) -> (w126:dynamicdata)
    n183 = Merge Signals(w163, w167) -> (w172:dynamicdata)
    "Waveform Chart 13" <- w172
    "Waveform Chart 12" <- w172
    n184 = Boolean To (0,1)(Boolean="Save Seq") -> (0, 1=w121:i16)
    n185 = for {
      N: w121 -> [_]
      tunnel: w126 -> [w407]
      tunnel: "Configuration file" -> [w408]
      tunnel: "Save Seq" -> [w406]
      n186 = call "Write To Measurement File2"("Signals"=w407, "Reset"=w406, "Filename"=w408) -> ()  [unwired: 14 in, 3 out]
    }
    n187 = call "STEPINDICATOR_091_4.vi"("current step"=w208, "enable"=i16 1, "manual"=w235) -> ("Led 8"=→"Led8 2":bool, "Led 10"=→"Led10 2":bool, "Led 11"=→"Led11 2":bool, "Led 7"=→"Led7 2":bool, "Led 1"=→"Led1 2":bool, "Led 6"=→"Led6 2":bool, "Led 2"=→"Led2 2":bool, "Led 12"=→"Led11 3":bool, "Led 5"=→"Led5 2":bool, "Led 4"=→"Led4 2":bool, "Led 3"=→"Led3 2":bool, "Led 9"=→"Led9 2":bool)  [unwired: 1 in]
    n188 = call "MWriteRS232_1.vi"("P3"=w117, "P2"=w118, "P1"=w119, "LAUDA"=w102) -> ()  [unwired: 8 in]
    n189 = Merge Signals(w173, w175, w172) -> (w171:dynamicdata)
    n190 = Boolean To (0,1)(Boolean="Read Seq") -> (0, 1=w120:i16)
    n191 = for {
      N: w120 -> [_]
      tunnel: "Configuration file" -> [w379]
      tunnel: "Read Seq" -> [w378]
      n192 = while {
        tunnel: [w405] -> w401
        tunnel: w379 -> [w404]
        tunnel: w378 -> [w402]
        stop <- w403 stop-if-true
        n193 = call "Read From Measurement File"("Filename"=w404, "Reset"=w402) -> ("Signals"=w405:dynamicdata, "EOF?"=w403:bool)  [unwired: 4 in, 4 out]
      }
      n194 = call "Convert from Dynamic Data"("Dynamic Data Type"=w401) -> ("Array"=w391:dbl[][])  [unwired: 3 in]
      "Config File" <- w391
      n195 = Array Subset(array=w391, index (row)=20 ("index"), length (row)=10 ("length")) -> (w398:dbl[][])  [unwired: 2 in]
      n196 = Array Subset(array=w391, index (row)=10 ("index"), length (row)=10 ("length")) -> (w393:dbl[][])  [unwired: 2 in]
      n197 = Array Subset(array=w391, index (row)=0 ("index"), length (row)=10 ("length")) -> (w392:dbl[][])  [unwired: 2 in]
      n198 = Array Subset(array=w391, index (row)=30 ("index"), length (row)=8 ("length")) -> (w380:dbl[][])  [unwired: 2 in]
      n199 = property on="PumpSeq 4" class="Arr (strict)"("Val(Sgnl)"=w398) -> ()  [unwired: 2 in, 2 out]
      n200 = property on="PumpSeq 2" class="Arr (strict)"("Val(Sgnl)"=w393) -> ()  [unwired: 2 in, 2 out]
      n201 = property on="PumpSeq 3" class="Arr (strict)"("Val(Sgnl)"=w392) -> ()  [unwired: 2 in, 2 out]
      n202 = Index Array(array=w380, index (row)=2, index (col)=0 ("disabled index (col)")) -> ()  [unwired: 1 out]
      n203 = Index Array(array=w380, index (row)=4, index (col)=0 ("disabled index (col)")) -> ()  [unwired: 1 out]
      n204 = Index Array(array=w380, index (row)=0, index (col)=1 ("disabled index (col)")) -> ()  [unwired: 1 out]
      n205 = Index Array(array=w380, index (row)=1, index (col)=1 ("disabled index (col)")) -> ()  [unwired: 1 out]
    }
    n206 = Merge Signals(w170, w171, w25) -> (w61:dynamicdata)
    n207 = call "Build Table"("Include time data"=TRUE, "Signals"=w61) -> ("Table"=w287:string[][])  [unwired: 3 in, 6 out]
    n208 = And(x="?", y="?") -> (x .and. y?=w14:bool)
    n209 = dll-call lib="C:/Users/shresplab/Desktop/Bertta-Bertta_deploy/Bertta-Bertta_deploy/BERTTA/x64/Debug/BERTTA.dll" fn="mettler"("port"="Scale port", "msg"=1) -> ("return type"=w7:dbl)  [unwired: 5 in, 2 out]
    n210 = And(x="MASTER CONTROL", y=w14) -> (x .and. y?=w10:bool)
    n211 = Initialize Array(FALSE, 1 ("dimension size")) -> (w12:bool[])
    n212 = Replace Array Subset(array=w12, new element=w10, index=0) -> (w9:bool[])
    n213 = call "Convert to Dynamic Data5"("Double"=w7) -> ("Dynamic Data Type"=→"Waveform Chart 15":dynamicdata)  [unwired: 3 in]
    n214 = Delete From Array(array=w287, length=13, index (col)=0 ("index (row)")) -> (array with subset deleted=→"Table":string[][])  [unwired: 1 in, 1 out]
    n215 = call "DAQ Assistant"("data"=w9, "device name"="PAM Control") -> ()  [unwired: 16 in, 2 out]
    n216 = call "filenameparser_09.vi"("Description"="Description", "start path"="Browse folder", "Project name"="Project name", "User (initials)"="User (initials)", "OK Button in"="OK Button 2") -> ("appended path 2"=w103:path, "appended path"=w283:path)  [unwired: 4 in, 1 out]
    "Output File" <- w103
    n217 = Boolean To (0,1)(Boolean="OK Button") -> (0, 1=w282:i16)
    n218 = for {
      N: w282 -> [_]
      tunnel: w283 -> [w370]
      w374 = " " ("string")
      n219 = property on="Add comment" class="Str"("Val(Sgnl)"="" ("Value (Signaling)")) -> ()  [unwired: 2 in, 2 out]
      n220 = Get Date/Time String(want seconds? (F)=TRUE) -> (date string=w377:string, time string=w375:string)  [unwired: 2 in]
      n221 = Concatenate Strings(w377, w374, w375, w374, "Add comment") -> (w373:string)
      n222 = feedback #8() -> (w372:string[])  [unwired: 1 in]
      n223 = Build Array (concatenate)(w372, w373) -> (w371:string[])
      n224 = feedback-in #8(w371) -> ()
      n225 = Write to Text File(file (use dialog)=w370, text=w371) -> ()  [unwired: 2 in, 3 out]
    }
    n226 = call "Header Names 4.vi"("Dynamic Data"=w61) -> ("Signals Out"=w62:dynamicdata)  [unwired: 10 in]
    n227 = call "Write To Measurement File"("Signals"=w62, "Enable"="OK Button 2", "Filename"=w103) -> ()  [unwired: 14 in, 3 out]
    "Boolean" <- "OK Button 2"
  }
